vi "BASE_Setting.vi"(8 "error in (no error)":errorcluster) -> (0 "error out":errorcluster)   [LabVIEW 2017]
doc: "this is Hardware setting to set ip address and com port of scanner"
uses:
  1eef56a0-abc2-489e-ba31-cff147ef0886.vi
  ea51104a-780c-477f-ba7f-f28da8f86296.vi
  7b8b5f90-77d1-4387-a868-400dd3d8bb0b.vi
  Global/PLC_to_Auto.vi
panel:
  in  "System Tab":T1(tab)
  in  "THREAD LOCKER ON OFF DELAY":dbl=1.0 min=1.0 max=30.0 step=0.1 format="%#.1g"
  in  "SET DELAY VALUE":bool
  in  "RESET NG":bool
  out "NG COUNTER":u16
  out "OK COUNTER":u16
  in  "RESET OK":bool
  in  "LH Scanner ip address":string
  in  "IP Address":string
  in  "Save Button":bool
  in  "Default Button":bool
  in  "RH Scanner Ip address":string
  in  "Back":bool
  # "BARCODE VERIFICATION SYSTEM REPORTS"
  # "Hardware Setting"
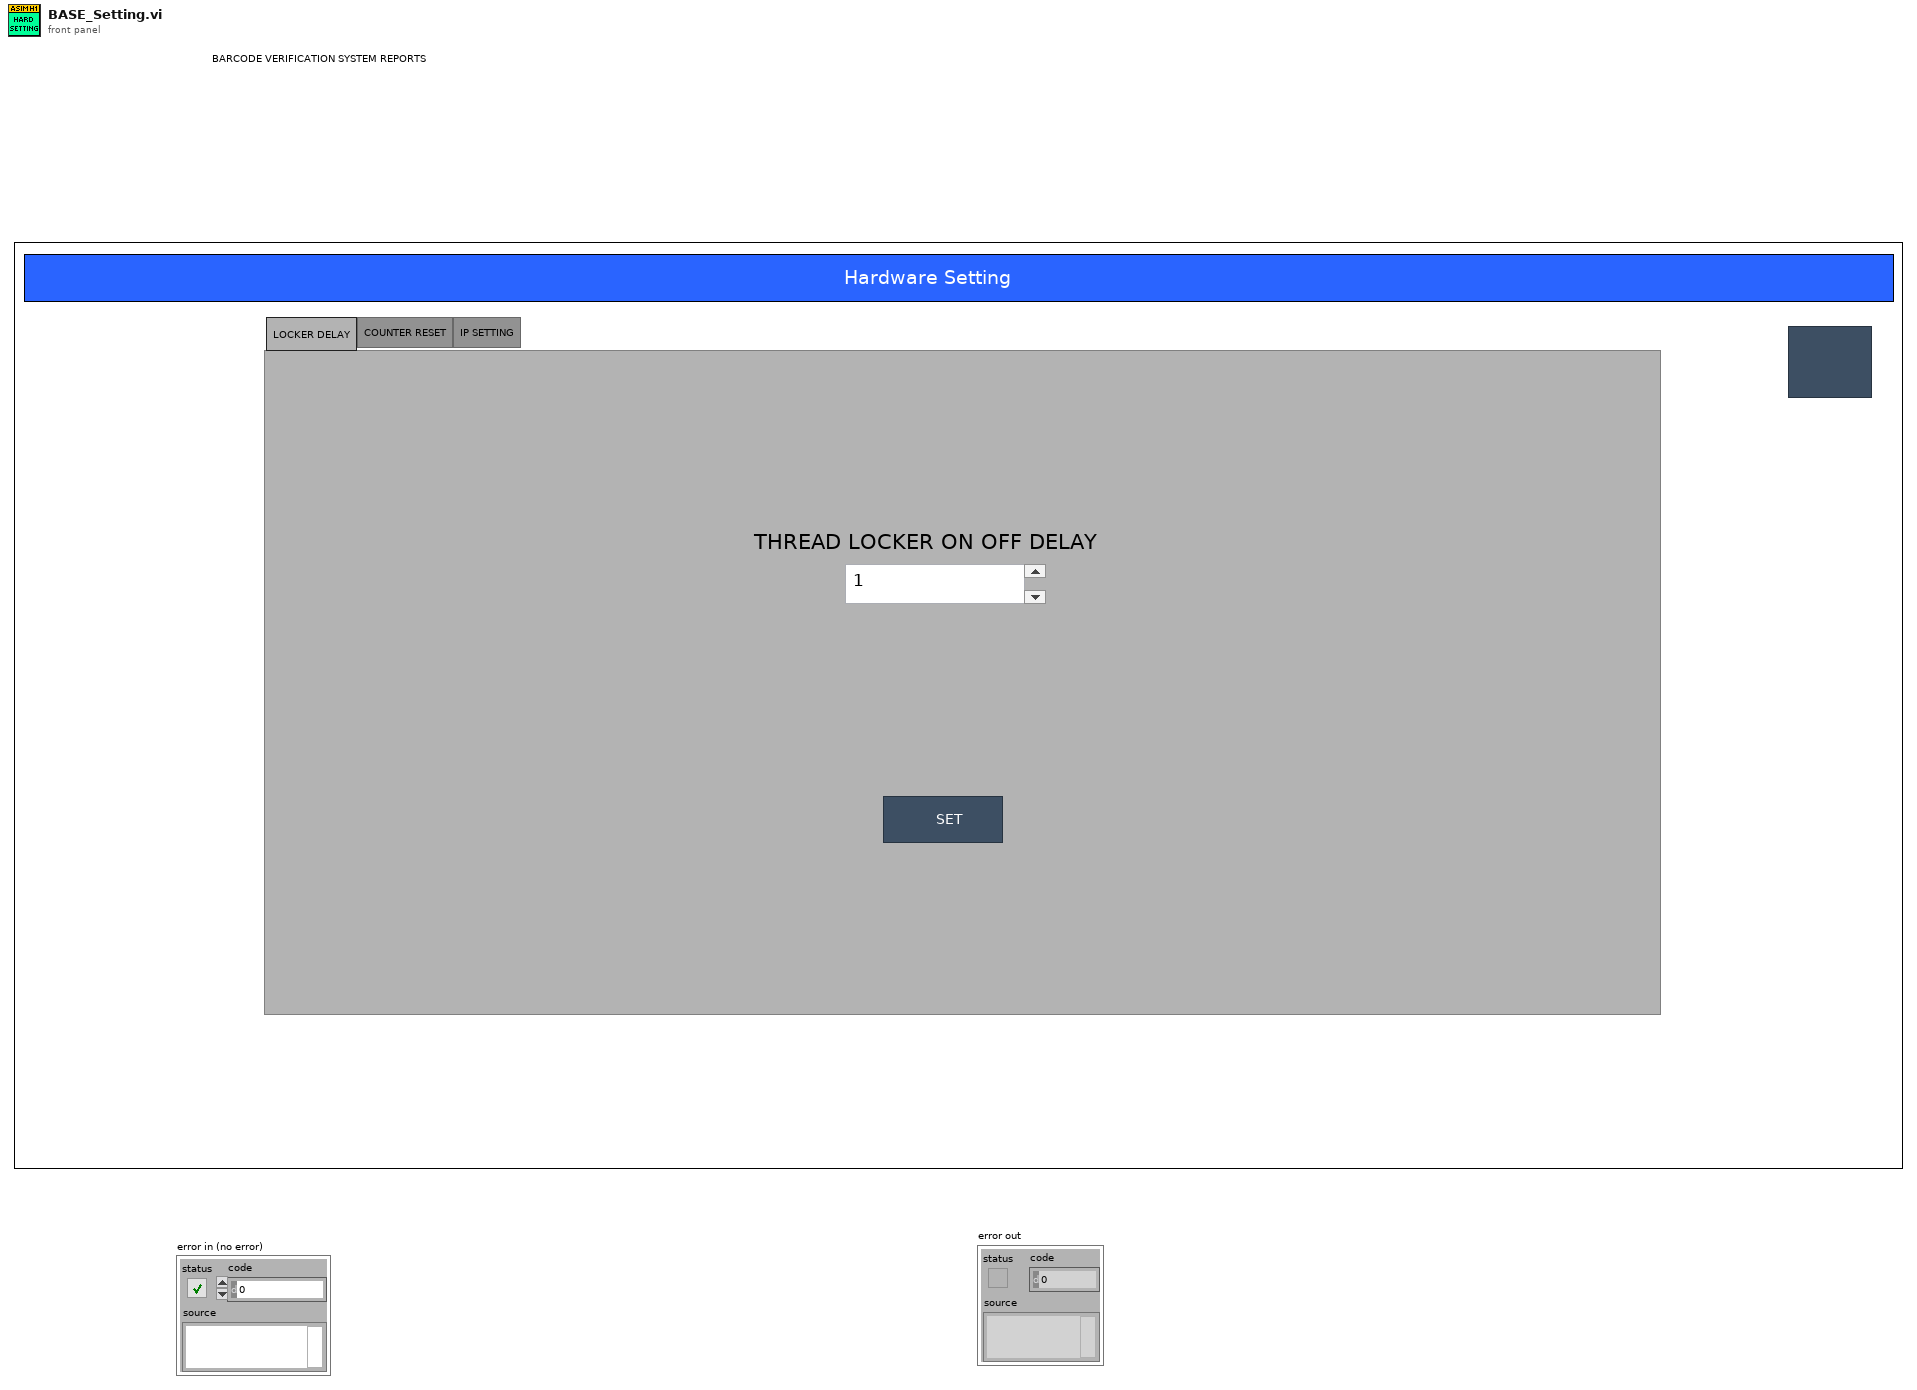
[diagram p1: front panel]
types:
  T1 = enum32{"LOCKER DELAY", "COUNTER RESET", "IP SETTING"}
  T2 = cluster{"IP Address":string, "LH Scanner IP Address":string, "RH Scanner IP Address":string}
  T3 = enum32{"invalid app kind", "Development System", "Run Time System", "Student Edition", "Embedded LabVIEW", "Evaluation", "Custom"}
  T4 = enum32{"Invalid", "Standard", "Closed", "Hidden", "Minimized", "Maximized"}
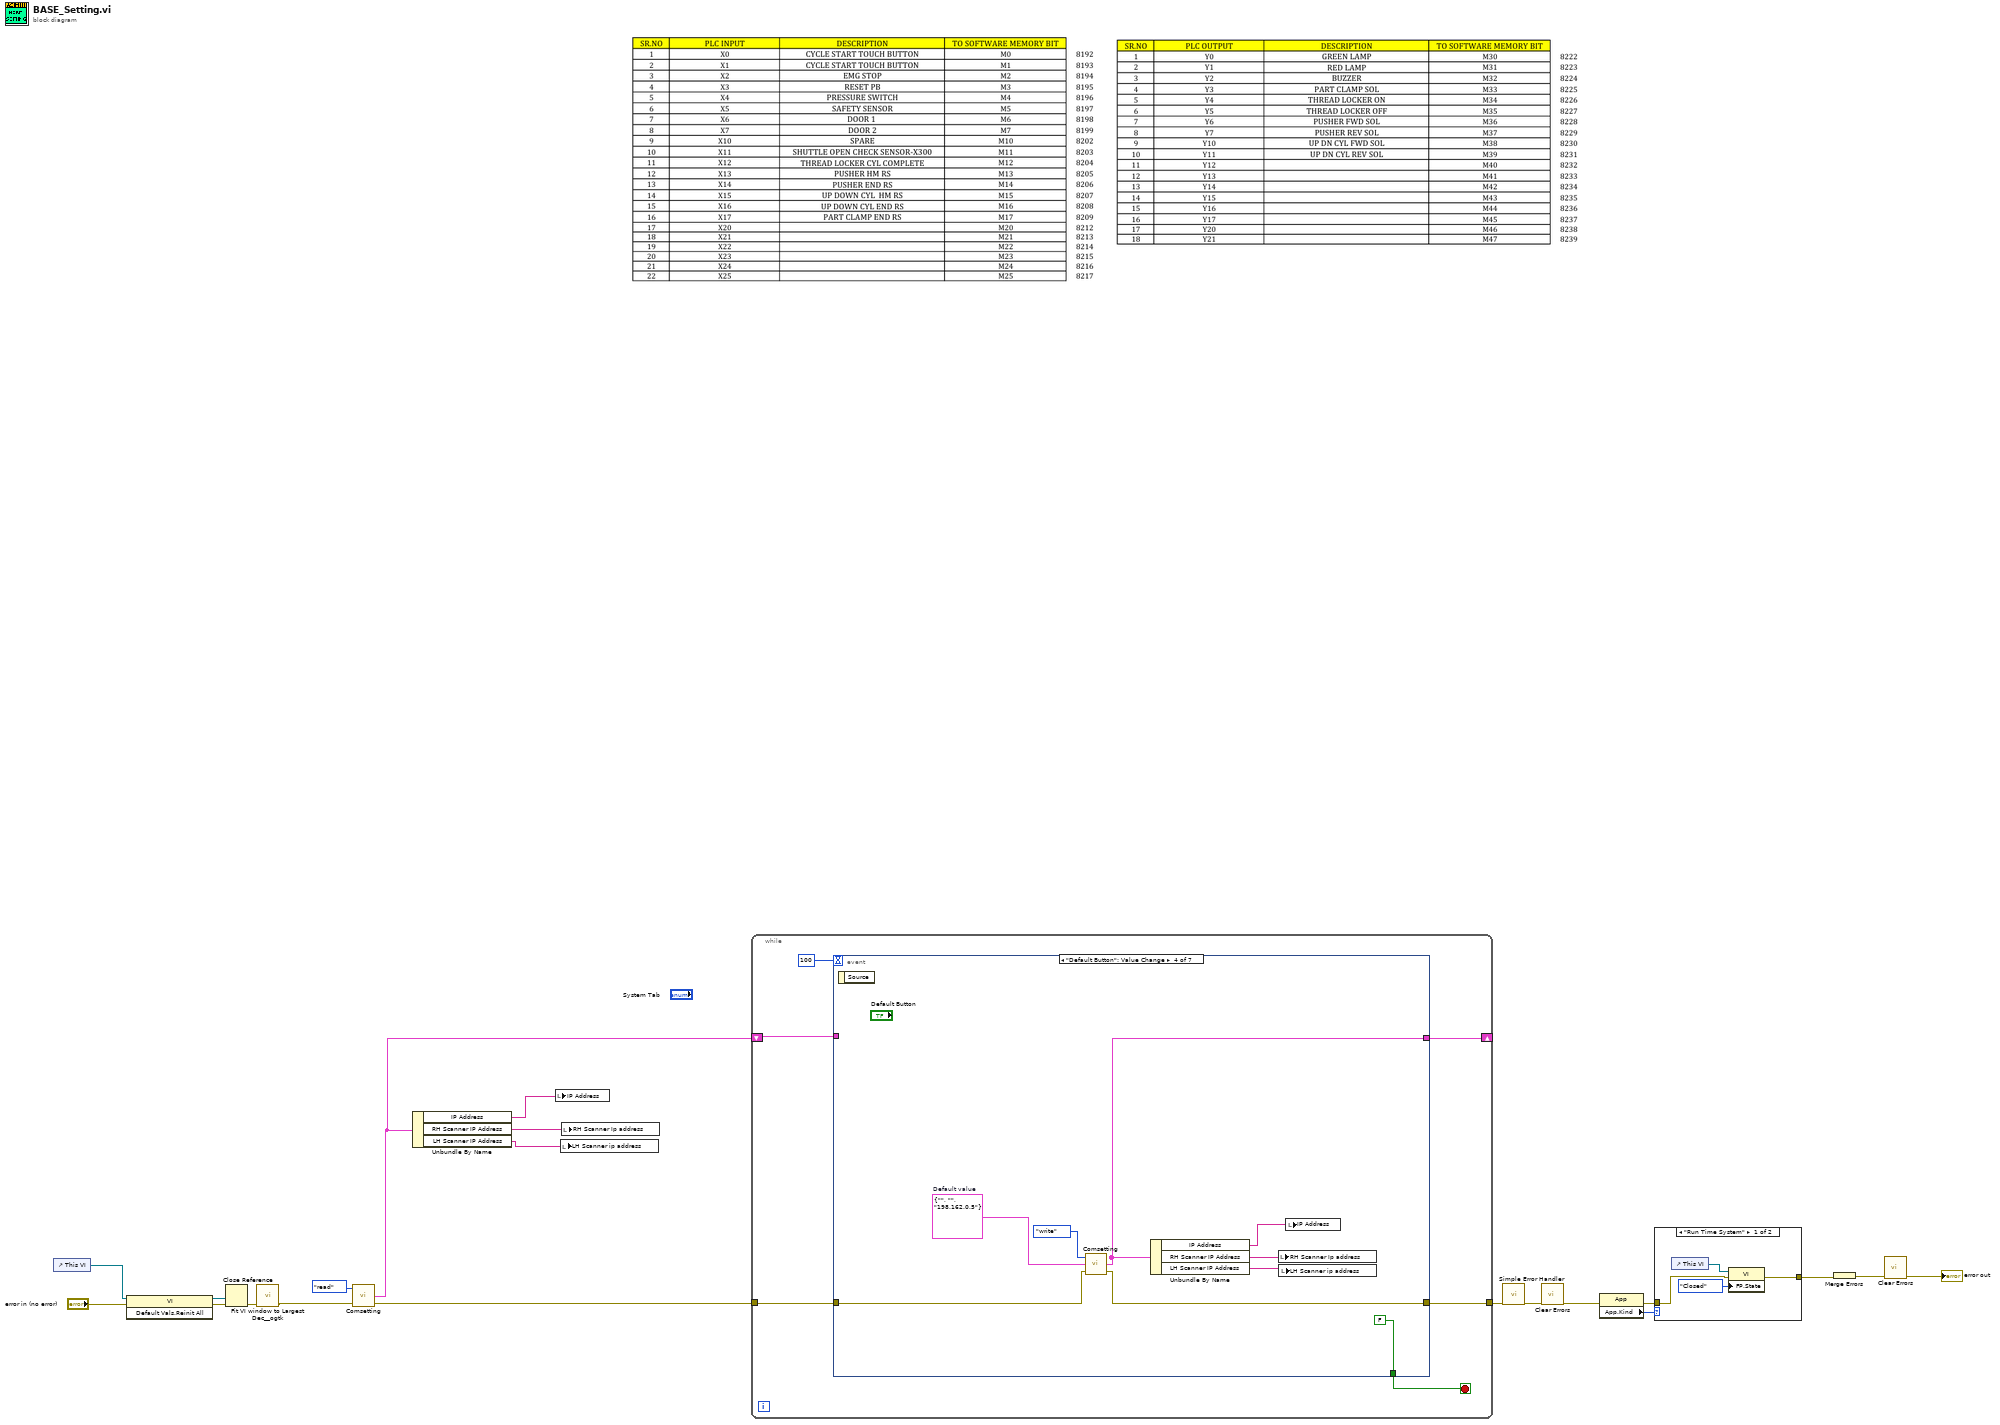
[diagram p0: block diagram]
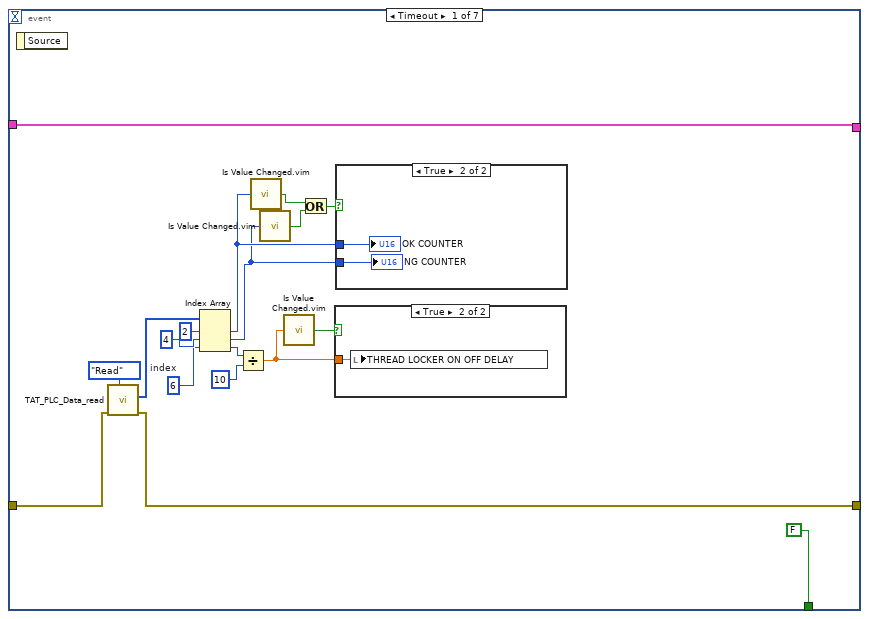
[diagram p2: hidden frame]
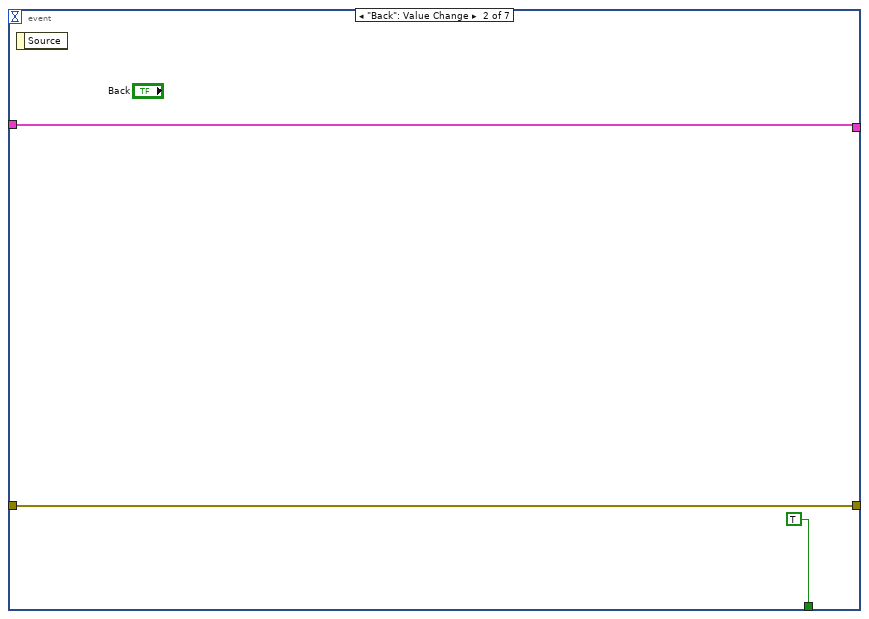
[diagram p5: hidden frame]
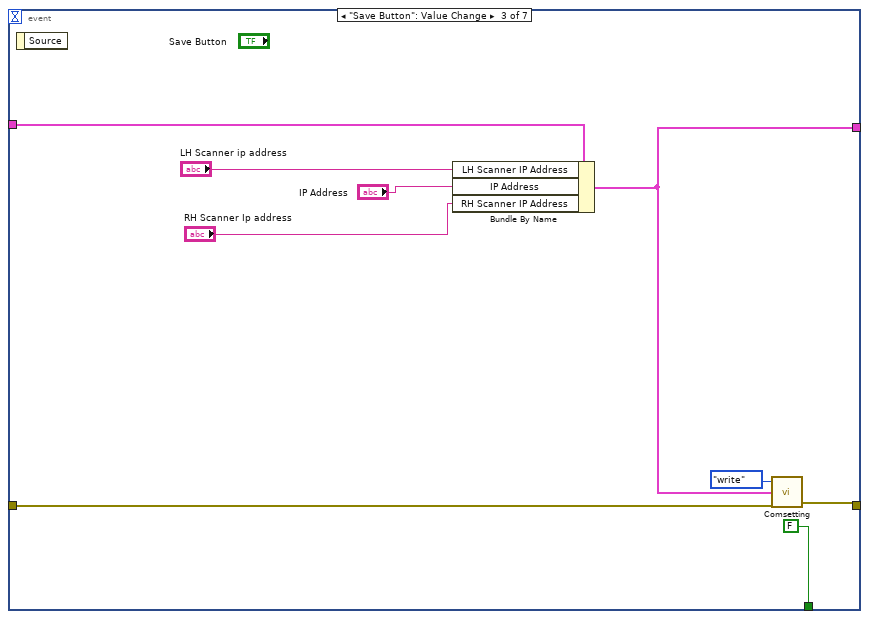
[diagram p6: hidden frame]
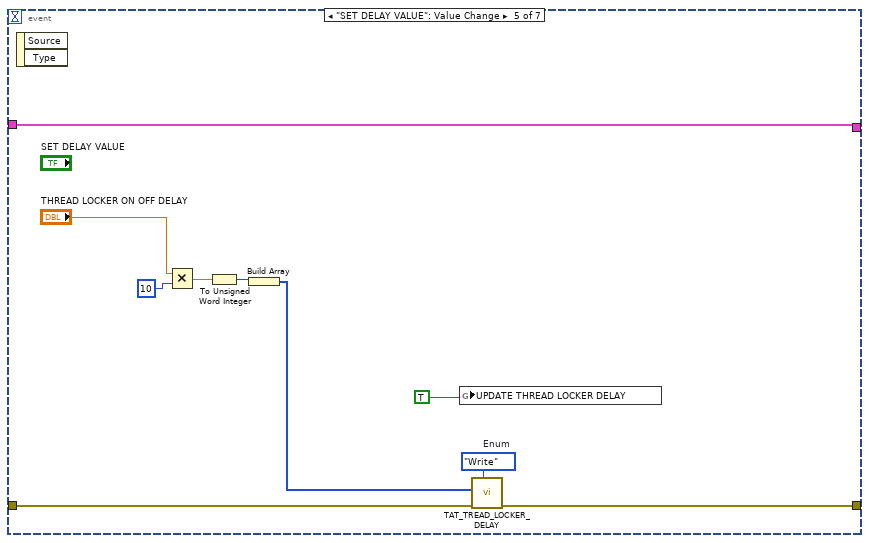
[diagram p7: hidden frame]
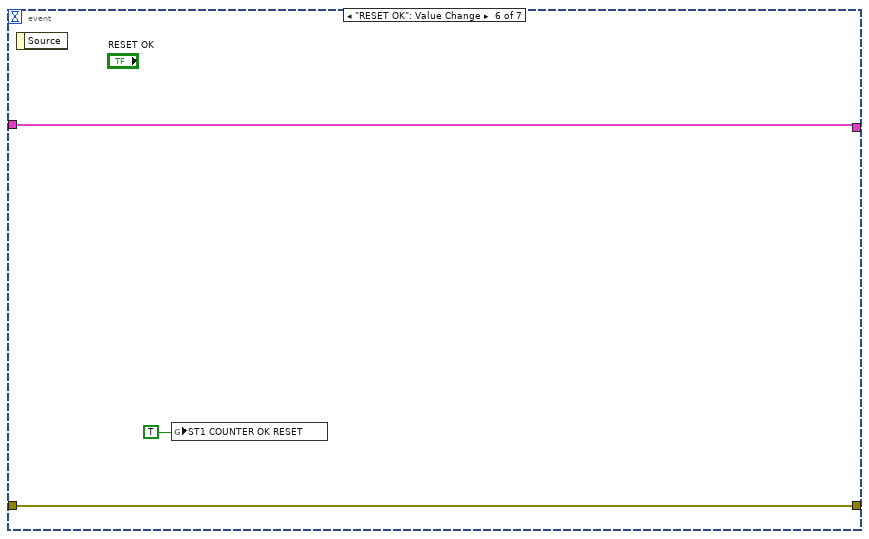
[diagram p8: hidden frame]
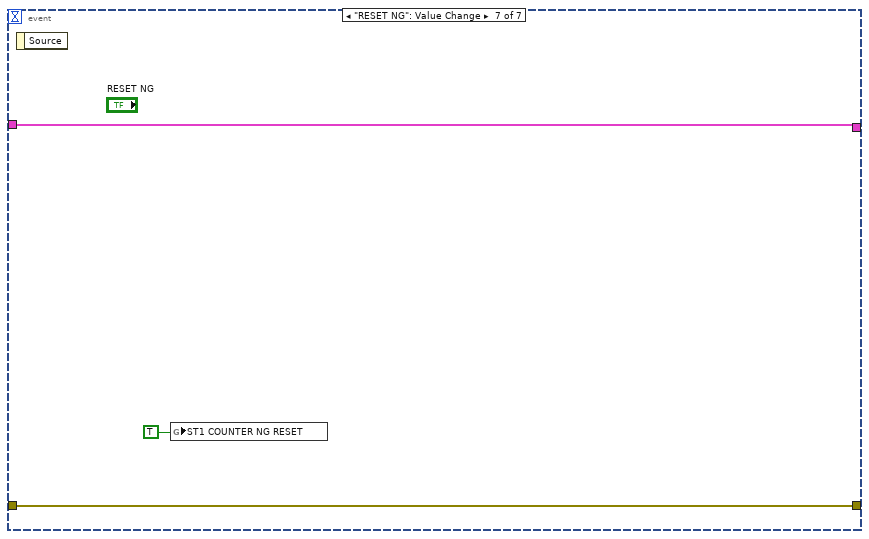
[diagram p9: hidden frame]
diagram:
  n1 = control-ref of="This VI"() -> (w17:refnum<vi>)
  n2 = invoke class="VI" method="Default Vals.Reinit All"(reference=w17, error in="error in (no error)") -> (reference out=w15:refnum<vi>, error out=w14:errorcluster)  [unwired: 1 in, 1 out]
  n3 = Close Reference(reference=w15, error in (no error)=w14) -> (error out=w13:errorcluster)
  n4 = call <userlib>:"Fit VI window to Largest Dec__ogtk.vi"("error in (no error)"=w13) -> ("error out"=w4:errorcluster)  [unwired: 5 in, 1 out]
  n5 = call "Comsetting.vi"("error in"=w4, "Enum"=enum16{"read", "write"}."read") -> ("error our"=w2:errorcluster, "Cluster Out"=w6:T2)  [unwired: 1 in, 1 out]
  n6 = Unbundle By Name(w6) -> ("IP Address"=w8:string, "RH Scanner IP Address"=w3:string, "LH Scanner IP Address"=w1:string)
  n7 = local write "IP Address"(w8) -> ()
  n8 = local write "LH Scanner ip address"(w1) -> ()
  n9 = local write "RH Scanner Ip address"(w3) -> ()
  n10 = while {
    tunnel: [w26] -> w5
    tunnel: w2 -> [w25]
    shift-right: [w24] -> _
    shift-left: w6 -> [w23]
    stop <- w21 stop-if-true
    n11 = event shown="[3] \"Default Button\": Value Change" {
      selector: _ -> [_ _ _ _ _ _ _]
      dyn-events: _ -> [_ _ _ _ _ _ _]
      timeout: 100 -> [_ _ _ _ _ _ _]
      tunnel: [w38 w49 w58 w67 w71 w81 w84] -> w26
      tunnel: w25 -> [w39 w49 w59 w68 w72 w81 w84]
      tunnel: w23 -> [w44 w48 w56 _ w78 w79 w82]
      tunnel: [w44 w48 w55 w65 w78 w79 w82] -> w24
      tunnel: [FALSE TRUE FALSE FALSE _ _ _] -> w21
      event Timeout {
        w33 = 6  # index
        n12 = event-data() -> ()  [unwired: 1 in, 1 out]
        n13 = call "TAT_PLC_Data_read.vi"("Enum"=enum16{"Read", "Write"}."Read", "error in (no error)"=w39) -> ("error out"=w38:errorcluster, "Array 2"=w42:u16[])  [unwired: 8 in]
        n14 = Index Array(array=w42, index #1=2 ("index"), index #2=4 ("index"), index #3=w33) -> (element #1=w28:u16, element #2=w27:u16, element #3=w32:u16)
        n15 = Divide(x=w32, y=10 ("Numeric 2")) -> (x/y=w36:dbl)
        n16 = call "Is Value Changed.vim"("value"=w28) -> ("changed or first call?"=w30:bool)
        n17 = call "Is Value Changed.vim"("value"=w27) -> ("changed or first call?"=w29:bool)
        n18 = call "Is Value Changed.vim"("value"=w36) -> ("changed or first call?"=w37:bool)
        n19 = Or(x=w30, y=w29) -> (x .or. y?=w31:bool)
        n20 = case shown="True" w37 {
          tunnel: w36 -> [_ w47]
          frame False {
          }
          frame True {
            n21 = local write "THREAD LOCKER ON OFF DELAY"(w47) -> ()
          }
        }
        n22 = case shown="True" w31 {
          tunnel: w28 -> [_ w46]
          tunnel: w27 -> [_ w45]
          frame False {
          }
          frame True {
            "NG COUNTER" <- w45
            "OK COUNTER" <- w46
          }
        }
      }
      event "Back": Value Change {
        n23 = event-data() -> ()  [unwired: 1 in, 1 out]
      }
      event "Save Button": Value Change {
        n24 = event-data() -> ()  [unwired: 1 in, 1 out]
        n25 = Bundle By Name(cluster=w56, "LH Scanner IP Address"="LH Scanner ip address", "IP Address"="IP Address", "RH Scanner IP Address"="RH Scanner Ip address") -> (w55:T2)
        n26 = call "Comsetting.vi"("error in"=w59, "Cluster In"=w55, "Enum"=enum16{"read", "write"}."write") -> ("error our"=w58:errorcluster)  [unwired: 2 out]
      }
      event "Default Button": Value Change {
        w60 = T2 {"IP Address"="", "LH Scanner IP Address"="", "RH Scanner IP Address"="198.162.0.5"}  # Default value
        n27 = event-data() -> ()  [unwired: 1 in, 1 out]
        n28 = call "Comsetting.vi"("error in"=w68, "Cluster In"=w60, "Enum"=enum16{"read", "write"}."write") -> ("error our"=w67:errorcluster, "Cluster Out"=w65:T2)  [unwired: 1 out]
        n29 = Unbundle By Name(w65) -> ("IP Address"=w64:string, "RH Scanner IP Address"=w62:string, "LH Scanner IP Address"=w61:string)
        n30 = local write "RH Scanner Ip address"(w62) -> ()
        n31 = local write "LH Scanner ip address"(w61) -> ()
        n32 = local write "IP Address"(w64) -> ()
      }
      event "SET DELAY VALUE": Value Change {
        w77 = enum16{"Read", "Write"}."Write"  # Enum
        n33 = event-data() -> ()  [unwired: 1 in, 2 out]
        n34 = Multiply(x="THREAD LOCKER ON OFF DELAY", y=10) -> (x*y=w74:dbl)
        n35 = To Unsigned Word Integer(number=w74) -> (unsigned 16bit integer=w73:u16)
        n36 = Build Array(w73) -> (w70:u16[])
        n37 = global write "PLC_to_Auto.vi" "UPDATE THREAD LOCKER DELAY"(TRUE) -> ()
        n38 = call "TAT_TREAD_LOCKER_DELAY.vi"("Enum"=w77, "error in (no error)"=w72, "Array"=w70) -> ("error out"=w71:errorcluster)  [unwired: 7 in, 1 out]
      }
      event "RESET OK": Value Change {
        n39 = event-data() -> ()  [unwired: 1 in, 1 out]
        n40 = global write "PLC_to_Auto.vi" "ST1 COUNTER OK RESET"(TRUE) -> ()
      }
      event "RESET NG": Value Change {
        n41 = event-data() -> ()  [unwired: 1 in, 1 out]
        n42 = global write "PLC_to_Auto.vi" "ST1 COUNTER NG RESET"(TRUE) -> ()
      }
    }
  }
  n43 = call <vilib>:"Simple Error Handler.vi"("error in (no error)"=w5) -> ("error out"=w12:errorcluster)  [unwired: 4 in, 4 out]
  n44 = call <vilib>:"Clear Errors.vi"("error in (no error)"=w12) -> ("error out"=w9:errorcluster)  [unwired: 5 in, 1 out]
  n45 = property class="App"(error in=w9) -> (error out=w10:errorcluster, "App.Kind"=w11:T3)  [unwired: 1 in, 1 out]
  n46 = case shown="\"Run Time System\"" w11 {
    tunnel: w10 -> [w86 w89]
    tunnel: [w85 w89] -> w18
    frame "Run Time System" {
      n47 = control-ref of="This VI"() -> (w88:refnum<vi>)
      n48 = property class="VI"(reference=w88, error in=w86, "FP.State"=T4."Closed" ("Front Panel Window:State")) -> (error out=w85:errorcluster)  [unwired: 1 out]
    }
    frame "Development System", Default {
    }
  }
  n49 = Merge Errors(w18) -> (w19:errorcluster)
  n50 = call <vilib>:"Clear Errors.vi"("error in (no error)"=w19) -> ("error out"=→"error out":errorcluster)  [unwired: 5 in, 1 out]
